vi "VI-Get XControl From Menu Launch.vi"(0 "Application in":refnum<vi>, 5 "App.MenuLaunchVI":string, 11 "error in (no error)":errorcluster) -> (4 "VI Path":path, 8 "Path":path, 10 "Found?":bool, 14 "Name":string, 15 "error out":errorcluster)   [LabVIEW 2015]
panel:
  out "Application out":refnum<vi>
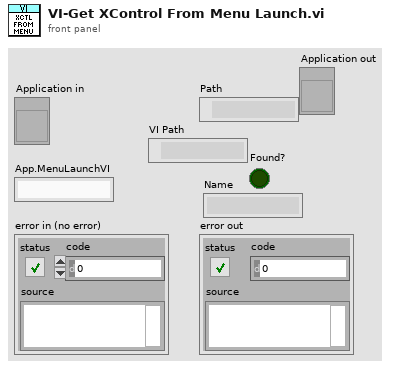
[diagram p1: front panel]
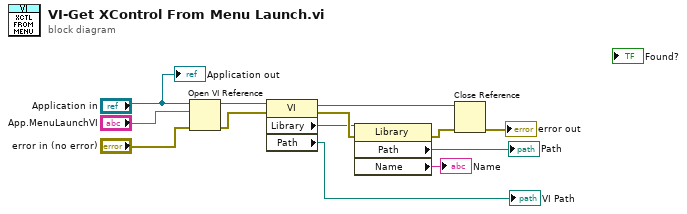
[diagram p0: block diagram]
diagram:
  n1 = Open VI Reference(application reference (local)="Application in", vi path="App.MenuLaunchVI", error in (no error)="error in (no error)") -> (vi reference=w5:refnum<vi>, error out=w6:errorcluster)  [unwired: 3 in]
  n2 = property class="VI"(reference=w5, error in=w6) -> (reference out=w10:refnum<vi>, error out=w8:errorcluster, "Library"=w7:refnum<vi>, "Path"=→"VI Path":path)
  n3 = property class="Library"(reference=w7, error in=w8) -> (error out=w9:errorcluster, "Path"=→"Path":path, "Name"=→"Name":string)  [unwired: 1 out]
  n4 = Close Reference(reference=w10, error in (no error)=w9) -> (error out=→"error out":errorcluster)
  "Application out" <- "Application in"
